vi "Parse JSON.vi"(8 "Path":string, 9 "Log File Ref":refnum<file>, 10 "Results In":refnum<class "Results.lvclass">, 11 "JSON Tree":variant) -> (3 "Results Out":refnum<class "Results.lvclass">)   [LabVIEW 2018, in "InfluxDB Client.lvlib" / "Client.lvclass"]
uses:
  Client.lvclass
  Results/Results.lvclass
  Results/Results.lvclass/Results.ctl
  Result/Result.lvclass/Result.ctl
  Series/Series.lvclass/Series.ctl
  <vilib>/LVH/i3 JSON/JSON Types/JSON Type.ctl
  Series/Series.lvclass
  Result/Result.lvclass
  Controls/TagSet.ctl
  <vilib>/LVH/i3 JSON/JSON Parsing/Get Array Value at Index Files/Get Array Value at Index - Object.vi
  <userlib>/_OpenG.lib/dictionary/dictionary.llb/Dictionary Create__ogtk.vi
  <userlib>/_OpenG.lib/dictionary/dictionary.llb/Dictionary Update__ogtk.vi
  <userlib>/_OpenG.lib/dictionary/dictionary.llb/Dictionary Update (by scalar value)__ogtk.vi
  <vilib>/LVH/i3 JSON/i3-json.lvlib
  InfluxDB Client.lvlib
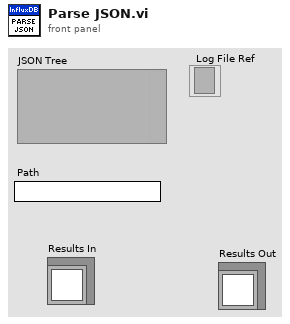
[diagram p1: front panel]
types:
  T1 = typedef "i3-json.lvlib/JSON Type.ctl" = enum8{"JSON Compatible", "JSON Array", "JSON Object", "JSON Null", "Double", "String", "Boolean", "Unknown"}
  T2 = typedef "InfluxDB Client.lvlib/TagSet.ctl" = cluster{"Key":string, "Value":string}
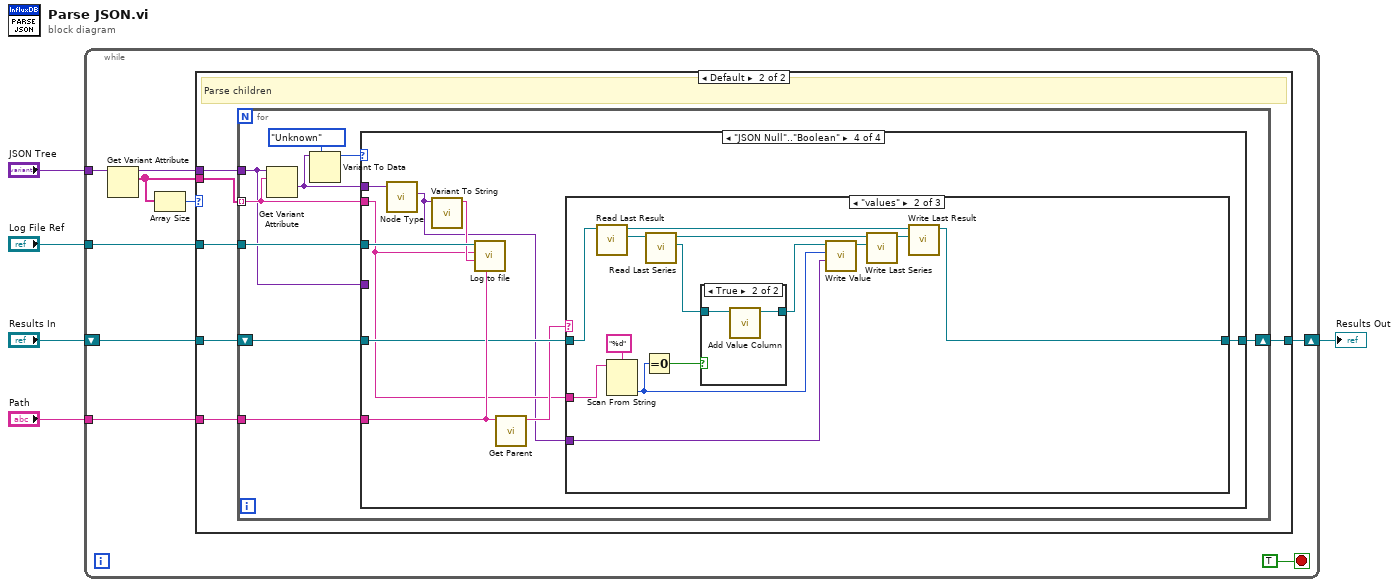
[diagram p0: block diagram]
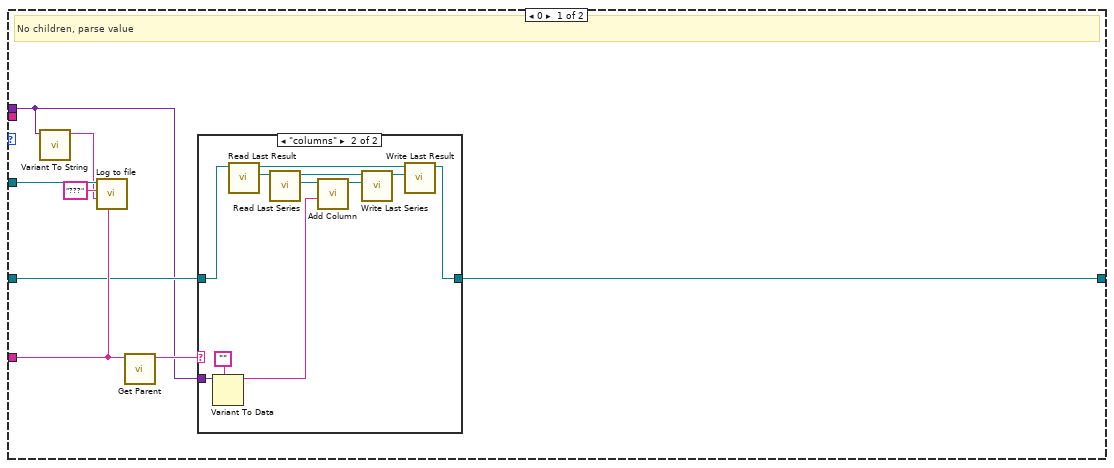
[diagram p2: hidden frame]
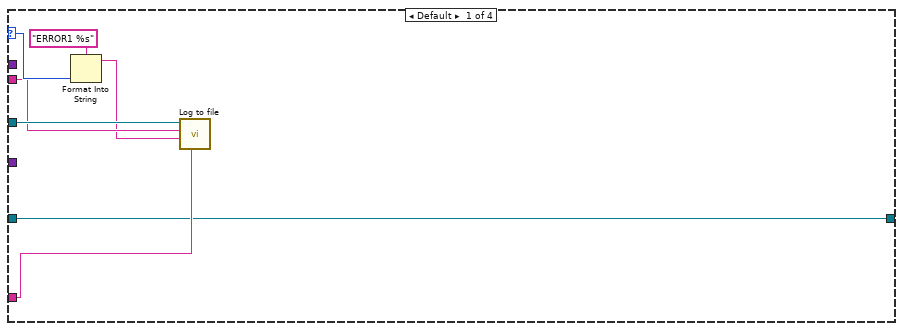
[diagram p4: hidden frame]
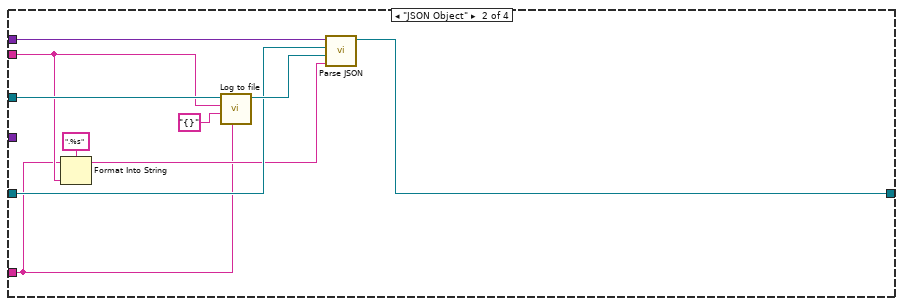
[diagram p5: hidden frame]
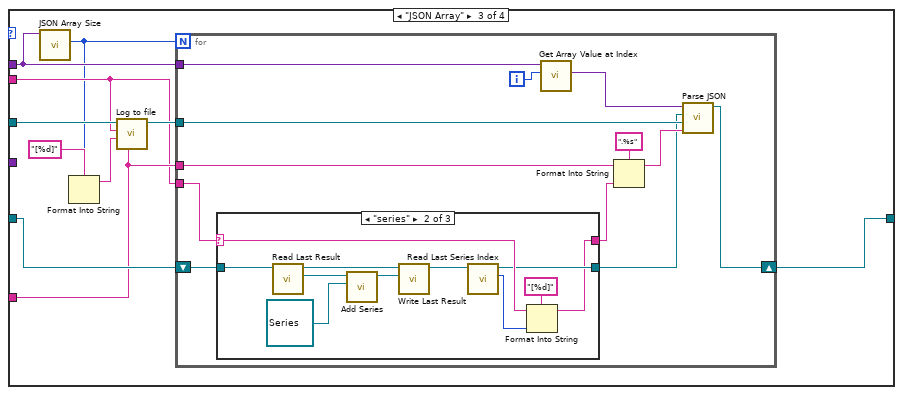
[diagram p6: hidden frame]
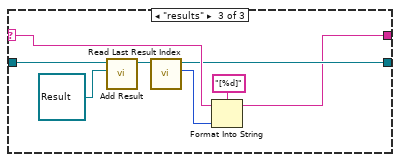
[diagram p8: hidden frame]
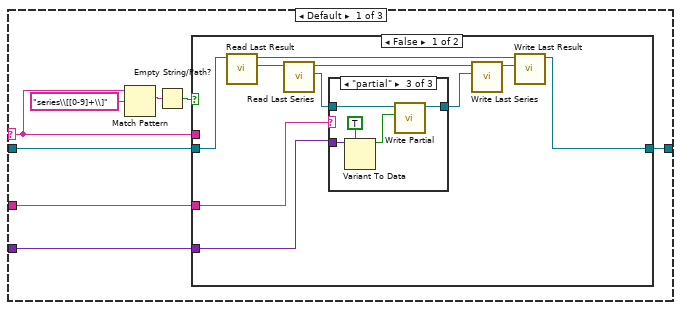
[diagram p9: hidden frame]
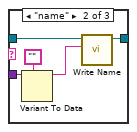
[diagram p11: hidden frame]
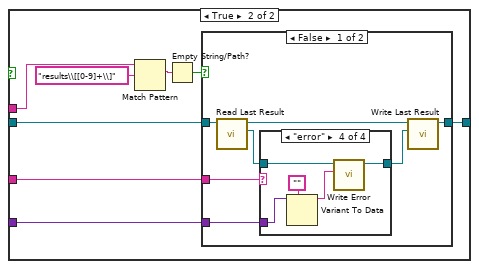
[diagram p12: hidden frame]
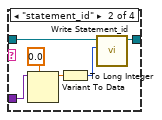
[diagram p14: hidden frame]
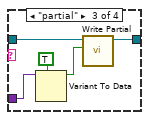
[diagram p15: hidden frame]
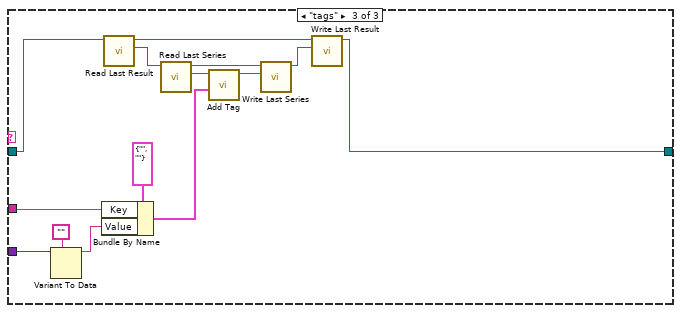
[diagram p18: hidden frame]
diagram:
  n1 = while {
    shift-right: [w10] -> w4
    shift-left: "Results In" -> [w11]
    tunnel: "Path" -> [w9]
    tunnel: "Log File Ref" -> [w8]
    tunnel: "JSON Tree" -> [w7]
    stop <- TRUE stop-if-true
    n2 = Get Variant Attribute(Variant=w7) -> (duplicate Variant=w14:variant, names=w12:string[])  [unwired: 3 in, 2 out]
    n3 = Array Size(array=w12) -> (size(s)=w13:i32)
    n4 = case shown="Default" w13 {
      tunnel: w12 -> [_ w40]
      tunnel: w14 -> [w16 w39]
      tunnel: w8 -> [w22 w38]
      tunnel: w11 -> [w19 w35]
      tunnel: w9 -> [w20 w37]
      tunnel: [w18 w36] -> w10
      frame 0 {
        # "No children, parse value"
        n5 = call "Variant To String.vi"("Variant"=w16) -> ("String"=w15:string)  [unwired: 9 in, 1 out]
        n6 = call "Log to file.vi"("path"=w20, "value"=w15, "name"="???", "Byte Stream File in"=w22) -> ()  [unwired: 7 in, 1 out]
        n7 = call "Get Parent.vi"("Path"=w20) -> ("parent"=w17:string)  [unwired: 10 in]
        n8 = case shown="\"columns\"" w17 {
          tunnel: w19 -> [w23 w34]
          tunnel: [w23 w29] -> w18
          tunnel: w16 -> [_ w25]
          frame Default {
          }
          frame "columns" {
            n9 = Variant To Data(type="", Variant=w25) -> (data=w24:string)  [unwired: 1 in, 1 out]
            n10 = call "Read Last Result.vi"("Results in"=w34) -> ("Result"=w33:refnum<class "Result.lvclass">, "Results out"=w31:refnum<class "Results.lvclass">)  [unwired: 9 in]
            n11 = call "Read Last Series.vi"("Result in"=w33) -> ("Series"=w28:refnum<class "Series.lvclass">, "Result out"=w32:refnum<class "Result.lvclass">)  [unwired: 9 in]
            n12 = call "Add Column.vi"(9:w24, "Series in"=w28) -> ("Series out"=w27:refnum<class "Series.lvclass">)  [unwired: 9 in]
            n13 = call "Write Last Series.vi"("Series"=w27, "Result in"=w32) -> ("Result out"=w30:refnum<class "Result.lvclass">)  [unwired: 9 in]
            n14 = call "Write Last Result.vi"("Result"=w30, "Results in"=w31) -> ("Results out"=w29:refnum<class "Results.lvclass">)  [unwired: 9 in]
          }
        }
      }
      frame Default {
        # "Parse children"
        n15 = for {
          tunnel: w39 -> [w44]
          tunnel: w40 -> [w46] mode=indexing
          tunnel: w38 -> [w45]
          tunnel: w37 -> [w41]
          shift-right: [w43] -> w36
          shift-left: w35 -> [w42]
          n16 = Get Variant Attribute(Variant=w44, name=w46) -> (value=w48:variant)  [unwired: 2 in, 3 out]
          n17 = Variant To Data(type=JSON_Type."Unknown" ("JSON Type"), Variant=w48) -> (data=w47:T1)  [unwired: 1 in, 1 out]
          n18 = case shown="\"JSON Null\"..\"Boolean\"" w47 {
            selector: w47 -> [w56 _ _ _]
            tunnel: w48 -> [_ w63 w76 w117]
            tunnel: w46 -> [w53 w59 w70 w111]
            tunnel: w45 -> [w54 w64 w75 w118]
            tunnel: w44 -> [_ _ _ _]
            tunnel: w42 -> [w50 w62 w73 w115]
            tunnel: w41 -> [w51 w57 w71 w116]
            tunnel: [w50 w61 w72 w114] -> w43
            frame Default {
              n19 = Format Into String(format string="ERROR1 %s", w56) -> (resulting string=w52:string)  [unwired: 2 in, 1 out]
              n20 = call "Log to file.vi"("path"=w51, "value"=w52, "name"=w53, "Byte Stream File in"=w54) -> ()  [unwired: 7 in, 1 out]
            }
            frame "JSON Object" {
              n21 = Format Into String(format string=".%s", initial string=w57, w59) -> (resulting string=w58:string)  [unwired: 1 in, 1 out]
              n22 = call "Log to file.vi"("path"=w57, "value"="{}", "name"=w59, "Byte Stream File in"=w64) -> ("Byte Stream File out"=w66:refnum<file>)  [unwired: 7 in]
              n23 = call "Parse JSON.vi"("Path"=w58, "Log File Ref"=w66, "Results In"=w62, "JSON Tree"=w63) -> ("Results Out"=w61:refnum<class "Results.lvclass">)  [unwired: 7 in]
            }
            frame "JSON Array" {
              n24 = call <vilib>:"JSON Array Size.vi"("JSON Tree In (JSON Array)"=w76) -> ("Array Size"=w68:i32)  [unwired: 8 in, 2 out]
              n25 = Format Into String(format string="[%d]", w68) -> (resulting string=w67:string)  [unwired: 2 in, 1 out]
              n26 = call "Log to file.vi"("path"=w71, "value"=w67, "name"=w70, "Byte Stream File in"=w75) -> ("Byte Stream File out"=w74:refnum<file>)  [unwired: 7 in]
              n27 = for {
                N: w68 -> [_]
                tunnel: w76 -> [w87]
                tunnel: w74 -> [w88]
                tunnel: w71 -> [w81]
                tunnel: w70 -> [w79]
                shift-right: [w82] -> w72
                shift-left: w73 -> [w80]
                i -> [w85]
                n28 = case shown="\"series\"" w79 {
                  selector: w79 -> [w89 w95 w105]
                  tunnel: w80 -> [w90 w101 w108]
                  tunnel: [w90 w93 w103] -> w78
                  tunnel: [w89 w92 w102] -> w77
                  frame Default {
                  }
                  frame "series" {
                    n29 = call "Read Last Result.vi"("Results in"=w101) -> ("Result"=w99:refnum<class "Result.lvclass">, "Results out"=w100:refnum<class "Results.lvclass">)  [unwired: 9 in]
                    n30 = call "Add Series.vi"("Series"=refnum<class "Series.lvclass"> refnum, "Result in"=w99) -> ("Result out"=w98:refnum<class "Result.lvclass">)  [unwired: 9 in]
                    n31 = call "Write Last Result.vi"("Result"=w98, "Results in"=w100) -> ("Results out"=w94:refnum<class "Results.lvclass">)  [unwired: 9 in]
                    n32 = call "Read Last Series Index.vi"("Results in"=w94) -> ("Series index"=w97:i32, "Results out"=w93:refnum<class "Results.lvclass">)  [unwired: 9 in]
                    n33 = Format Into String(format string="[%d]", initial string=w95, w97) -> (resulting string=w92:string)  [unwired: 1 in, 1 out]
                  }
                  frame "results" {
                    n34 = call "Add Result.vi"("Result"=refnum<class "Result.lvclass"> refnum ("Result.lvclass"), "Results in"=w108) -> ("Results out"=w104:refnum<class "Results.lvclass">)  [unwired: 8 in, 1 out]
                    n35 = call "Read Last Result Index.vi"("Results in"=w104) -> ("Result index"=w107:i32, "Results out"=w103:refnum<class "Results.lvclass">)  [unwired: 9 in]
                    n36 = Format Into String(format string="[%d]", initial string=w105, w107) -> (resulting string=w102:string)  [unwired: 1 in, 1 out]
                  }
                }
                n37 = call-poly <vilib>:"Get Array Value at Index.vi"("Index"=w85, "JSON Tree In (JSON Array)"=w87) -> ("JSON Object"=w86:variant)  [unwired: 6 in, 3 out]
                n38 = Format Into String(format string=".%s", initial string=w81, w77) -> (resulting string=w83:string)  [unwired: 1 in, 1 out]
                n39 = call "Parse JSON.vi"("Path"=w83, "Log File Ref"=w88, "Results In"=w78, "JSON Tree"=w86) -> ("Results Out"=w82:refnum<class "Results.lvclass">)  [unwired: 7 in]
              }
            }
            frame "JSON Null".."Boolean" {
              n40 = call <vilib>:"Node Type.vi"("JSON Tree In"=w117) -> ("Value"=w110:variant)  [unwired: 6 in, 4 out]
              n41 = call "Variant To String.vi"("Variant"=w110) -> ("String"=w112:string)  [unwired: 9 in, 1 out]
              n42 = call "Log to file.vi"("path"=w116, "value"=w112, "name"=w111, "Byte Stream File in"=w118) -> ()  [unwired: 7 in, 1 out]
              n43 = call "Get Parent.vi"("Path"=w116) -> ("parent"=w113:string)  [unwired: 10 in]
              n44 = case shown="\"values\"" w113 {
                selector: w113 -> [w120 _ _]
                tunnel: w115 -> [w125 w194 w211]
                tunnel: w111 -> [w123 w188 w204]
                tunnel: [w124 w189 w206] -> w114
                tunnel: w110 -> [w119 w184 w200]
                frame Default {
                  n45 = Match Pattern(string=w120, regular expression="series\\[[0-9]+\\]") -> (match substring=w121:string)  [unwired: 1 in, 3 out]
                  n46 = Empty String/Path?(string/path=w121) -> (empty?=w122:bool)
                  n47 = case shown="False" w122 {
                    tunnel: w125 -> [w131 w151]
                    tunnel: [w130 w150] -> w124
                    tunnel: w123 -> [w129 w149]
                    tunnel: w120 -> [_ w153]
                    tunnel: w119 -> [w127 w148]
                    frame False {
                      n48 = call "Read Last Result.vi"("Results in"=w131) -> ("Result"=w136:refnum<class "Result.lvclass">, "Results out"=w133:refnum<class "Results.lvclass">)  [unwired: 9 in]
                      n49 = call "Read Last Series.vi"("Result in"=w136) -> ("Series"=w135:refnum<class "Series.lvclass">, "Result out"=w134:refnum<class "Result.lvclass">)  [unwired: 9 in]
                      n50 = case shown="\"partial\"" w129 {
                        tunnel: w135 -> [w137 w142 w147]
                        tunnel: w127 -> [_ w138 w144]
                        tunnel: [w137 w141 w146] -> w128
                        frame Default {
                        }
                        frame "name" {
                          n51 = Variant To Data(type="", Variant=w138) -> (data=w139:string)  [unwired: 1 in, 1 out]
                          n52 = call "Write Name.vi"("Name"=w139, "Series in"=w142) -> ("Series out"=w141:refnum<class "Series.lvclass">)  [unwired: 9 in]
                        }
                        frame "partial" {
                          n53 = Variant To Data(type=TRUE, Variant=w144) -> (data=w143:bool)  [unwired: 1 in, 1 out]
                          n54 = call "Write Partial.vi"("Partial"=w143, "Series in"=w147) -> ("Series out"=w146:refnum<class "Series.lvclass">)  [unwired: 9 in]
                        }
                      }
                      n55 = call "Write Last Series.vi"("Series"=w128, "Result in"=w134) -> ("Result out"=w132:refnum<class "Result.lvclass">)  [unwired: 9 in]
                      n56 = call "Write Last Result.vi"("Result"=w132, "Results in"=w133) -> ("Results out"=w130:refnum<class "Results.lvclass">)  [unwired: 9 in]
                    }
                    frame True {
                      n57 = Match Pattern(string=w153, regular expression="results\\[[0-9]+\\]") -> (match substring=w155:string)  [unwired: 1 in, 3 out]
                      n58 = Empty String/Path?(string/path=w155) -> (empty?=w152:bool)
                      n59 = case shown="False" w152 {
                        tunnel: w151 -> [w159 w180]
                        tunnel: [w158 w180] -> w150
                        tunnel: w149 -> [w157 _]
                        tunnel: w148 -> [w156 _]
                        frame False {
                          n60 = call "Read Last Result.vi"("Results in"=w159) -> ("Result"=w161:refnum<class "Result.lvclass">, "Results out"=w162:refnum<class "Results.lvclass">)  [unwired: 9 in]
                          n61 = case shown="\"error\"" w157 {
                            tunnel: w161 -> [w163 w169 w174 w179]
                            tunnel: w156 -> [_ w166 w171 w176]
                            tunnel: [w163 w168 w173 w178] -> w160
                            frame Default {
                            }
                            frame "statement_id" {
                              n62 = Variant To Data(type=0.0, Variant=w166) -> (data=w165:dbl)  [unwired: 1 in, 1 out]
                              n63 = To Long Integer(number=w165) -> (32bit integer=w164:i32)
                              n64 = call "Write Statement_id.vi"("Statement_id"=w164, "Result in"=w169) -> ("Result out"=w168:refnum<class "Result.lvclass">)  [unwired: 9 in]
                            }
                            frame "partial" {
                              n65 = Variant To Data(type=TRUE, Variant=w171) -> (data=w170:bool)  [unwired: 1 in, 1 out]
                              n66 = call "Write Partial.vi"("Partial"=w170, "Result in"=w174) -> ("Result out"=w173:refnum<class "Result.lvclass">)  [unwired: 9 in]
                            }
                            frame "error" {
                              n67 = Variant To Data(type="", Variant=w176) -> (data=w175:string)  [unwired: 1 in, 1 out]
                              n68 = call "Write Error.vi"("Error"=w175, "Result in"=w179) -> ("Result out"=w178:refnum<class "Result.lvclass">)  [unwired: 9 in]
                            }
                          }
                          n69 = call "Write Last Result.vi"("Result"=w160, "Results in"=w162) -> ("Results out"=w158:refnum<class "Results.lvclass">)  [unwired: 9 in]
                        }
                        frame True {
                        }
                      }
                    }
                  }
                }
                frame "values" {
                  n70 = call "Read Last Result.vi"("Results in"=w194) -> ("Result"=w193:refnum<class "Result.lvclass">, "Results out"=w191:refnum<class "Results.lvclass">)  [unwired: 9 in]
                  n71 = Scan From String(format string="%d", input string=w188) -> (output 1=w181:i32)  [unwired: 3 in, 3 out]
                  n72 = Equal To 0?(x=w181) -> (x = 0?=w186:bool)
                  n73 = call "Read Last Series.vi"("Result in"=w193) -> ("Series"=w182:refnum<class "Series.lvclass">, "Result out"=w192:refnum<class "Result.lvclass">)  [unwired: 9 in]
                  n74 = case shown="True" w186 {
                    tunnel: w182 -> [w195 w197]
                    tunnel: [w195 w196] -> w185
                    frame False {
                    }
                    frame True {
                      n75 = call "Add Value Column.vi"("Series in"=w197) -> ("Series out"=w196:refnum<class "Series.lvclass">)  [unwired: 10 in]
                    }
                  }
                  n76 = call "Write Value.vi"("Variant"=w184, "Row"=w181, "Series in"=w185) -> ("Series out"=w183:refnum<class "Series.lvclass">)  [unwired: 8 in]
                  n77 = call "Write Last Series.vi"("Series"=w183, "Result in"=w192) -> ("Result out"=w190:refnum<class "Result.lvclass">)  [unwired: 9 in]
                  n78 = call "Write Last Result.vi"("Result"=w190, "Results in"=w191) -> ("Results out"=w189:refnum<class "Results.lvclass">)  [unwired: 9 in]
                }
                frame "tags" {
                  n79 = Variant To Data(type="", Variant=w200) -> (data=w198:string)  [unwired: 1 in, 1 out]
                  n80 = Bundle By Name(cluster=T2 {"Key"="", "Value"=""} ("TagSet"), "Key"=w204, "Value"=w198) -> (w202:T2)
                  n81 = call "Read Last Result.vi"("Results in"=w211) -> ("Result"=w210:refnum<class "Result.lvclass">, "Results out"=w208:refnum<class "Results.lvclass">)  [unwired: 9 in]
                  n82 = call "Read Last Series.vi"("Result in"=w210) -> ("Series"=w205:refnum<class "Series.lvclass">, "Result out"=w209:refnum<class "Result.lvclass">)  [unwired: 9 in]
                  n83 = call "Add Tag.vi"("TagSet"=w202, "Series in"=w205) -> ("Series out"=w201:refnum<class "Series.lvclass">)  [unwired: 9 in]
                  n84 = call "Write Last Series.vi"("Series"=w201, "Result in"=w209) -> ("Result out"=w207:refnum<class "Result.lvclass">)  [unwired: 9 in]
                  n85 = call "Write Last Result.vi"("Result"=w207, "Results in"=w208) -> ("Results out"=w206:refnum<class "Results.lvclass">)  [unwired: 9 in]
                }
              }
            }
          }
        }
      }
    }
  }
  "Results Out" <- w4
